vi "Test Log Error Message.vi"(8 "error in (no error)":errorcluster, 11 "Test Case In":refnum<class "Logger Test.lvclass">) -> (0 "error out":errorcluster, 3 "Test Case Out":refnum<class "Logger Test.lvclass">)   [LabVIEW 2020, in "Logger Test.lvclass"]
uses:
  Logger Test.lvclass
  C:/Program Files (x86)/National Instruments/LabVIEW 2020/vi.lib/Asteme/LUnit/Test Case.lvclass
  Mock Process/Mock Process.lvclass
  C:/Users/anton/Documents/GitHub/Triarc-Framework/source/Framework/Process/Process.lvclass
  C:/Users/anton/Documents/GitHub/Triarc-Framework/source/Framework/Logging/Logging.lvclass
  Mock Log Handler/Mock Log Handler.lvclass
  <vilib>/Asteme/LUnit/Test Case.lvclass/Test Case.ctl
  <vilib>/Asteme/LUnit/LUnit Assertion Result.lvclass/LUnit Assertion Result.ctl
  <vilib>/Asteme/LUnit/Palette/Pass.vi
  <vilib>/Asteme/LUnit/Palette/Fail.vi
  <vilib>/Asteme/LUnit/Variant to string.vi
  <vilib>/Asteme/LUnit/Set Assertion Type.vi
  <vilib>/Asteme/LUnit/Add test result.vi
  <vilib>/Asteme/LUnit/LUnit Write Passed.vi
  <vilib>/Asteme/LUnit/LUnit Get Test Case.vi
  <vilib>/Asteme/LUnit/LUnit Write Message.vi
  <vilib>/Asteme/LUnit/LUnit Write Description.vi
  <vilib>/Asteme/LUnit/LUnit Write Assertion Type.vi
  <vilib>/Asteme/LUnit/Read Test Case Name.vi
  <vilib>/Asteme/LUnit/Assertion Result/LUnit Get Test Name.vi
  <vilib>/Utility/Data Type/Get Type Information.vi
  <vilib>/Utility/LVClass/Get LV Class Name.vi
  <vilib>/Asteme/LUnit/LUnit Assertion Result.lvclass
  Framework/Process/Process.lvclass
  <vilib>/Asteme/LUnit/Test Case.lvclass
  Framework/Logging/Logging.lvclass
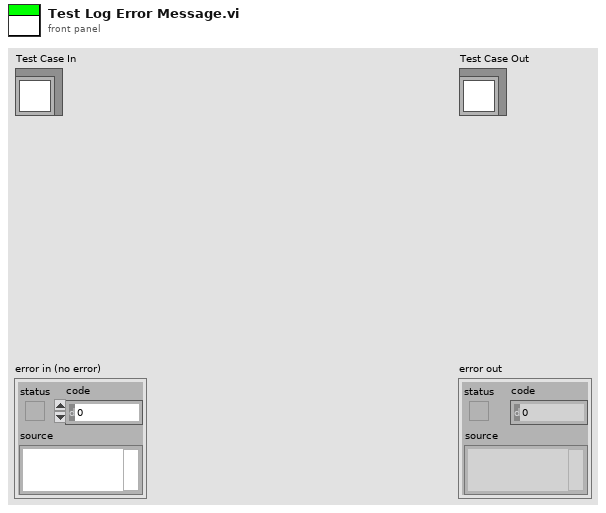
[diagram p1: front panel]
types:
  T1 = typedef "Mock Log Handler.lvclass/Log Entry.ctl" = cluster{"Level":string, "Source":string, "Message":string}
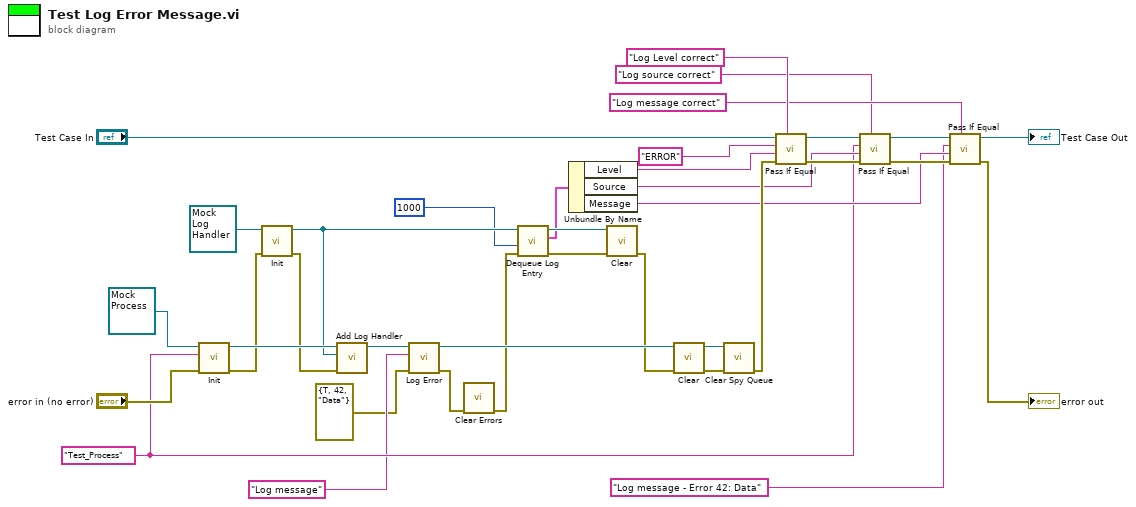
[diagram p0: block diagram]
diagram:
  w6 = "Test_Process" ("Name")
  n1 = call-dynamic "Init.vi"("error in (no error)"="error in (no error)", "Name"=w6, "Mock Process In"=refnum<class "Mock Process.lvclass"> refnum) -> ("error out"=w28:errorcluster, "Mock Process Out"=w34:refnum<class "Mock Process.lvclass">)  [unwired: 7 in]
  n2 = call-dynamic "Init.vi"("error in (no error)"=w28, "Mock Log Handler In"=refnum<class "Mock Log Handler.lvclass"> refnum ("Mock Log Handler.lvclass")) -> ("error out"=w27:errorcluster, "Mock Log Handler Out"=w24:refnum<class "Mock Log Handler.lvclass">)  [unwired: 8 in]
  n3 = call "Add Log Handler.vi"("error in (no error)"=w27, "Log Handler"=w24, "Process In"=w34) -> ("Process Out"=w22:refnum<class "Mock Process.lvclass">)  [unwired: 7 in, 1 out]
  n4 = call "Log Error.vi"("error in (no error)"=errorcluster {"status"=TRUE, "code"=42, "source"="Data"}, "Message"="Log message", "Logging In"=w22) -> ("error out"=w3:errorcluster, "Logging Out"=w21:refnum<class "Mock Process.lvclass">)  [unwired: 7 in]
  n5 = call <vilib>:"Clear Errors.vi"("error in (no error)"=w3) -> ("error out"=w2:errorcluster)  [unwired: 5 in, 1 out]
  n6 = call "Dequeue Log Entry.vi"("error in (no error)"=w2, "timeout in ms (-1)"=1000, "Mock Log Handler in"=w24) -> ("error out"=w25:errorcluster, "Entry"=w19:T1, "Mock Log Handler out"=w26:refnum<class "Mock Log Handler.lvclass">)  [unwired: 5 in, 1 out]
  n7 = Unbundle By Name(w19) -> ("Level"=w18:string, "Source"=w8:string, "Message"=w7:string)
  n8 = call-dynamic "Clear.vi"("error in (no error)"=w25, "Mock Log Handler In"=w26) -> ("error out"=w20:errorcluster)  [unwired: 8 in, 1 out]
  n9 = call-dynamic "Clear.vi"("error in (no error)"=w20, "Mock Process In"=w21) -> ("error out"=w32:errorcluster, "Mock Process Out"=w33:refnum<class "Mock Process.lvclass">)  [unwired: 8 in]
  n10 = call-dynamic "Clear Spy Queue.vi"("error in (no error)"=w32, "Mock Process In"=w33) -> ("error out"=w12:errorcluster)  [unwired: 8 in, 1 out]
  n11 = call <vilib>:"Pass If Equal.vi"("Description"="Log Level correct", "error in (no error)"=w12, "Actual"=w18, "Expected"="ERROR", "Test Case In"="Test Case In") -> ("error out"=w14:errorcluster, "Test Case Out"=w36:refnum<class "Logger Test.lvclass">)  [unwired: 5 in]
  n12 = call <vilib>:"Pass If Equal.vi"("Description"="Log source correct", "error in (no error)"=w14, "Actual"=w8, "Expected"=w6, "Test Case In"=w36) -> ("error out"=w13:errorcluster, "Test Case Out"=w16:refnum<class "Logger Test.lvclass">)  [unwired: 5 in]
  n13 = call <vilib>:"Pass If Equal.vi"("Description"="Log message correct", "error in (no error)"=w13, "Actual"=w7, "Expected"="Log message - Error 42: Data" ("Message"), "Test Case In"=w16) -> ("error out"=→"error out":errorcluster, "Test Case Out"=→"Test Case Out":refnum<class "Logger Test.lvclass">)  [unwired: 5 in]
